vi "Setup.vi"(11 "Network Session Handler in":refnum<class "Network Session Handler.lvclass">) -> (0 "error out":errorcluster, 3 "Network Session Handler out":refnum<class "Network Session Handler.lvclass">)   [LabVIEW 2017, in "Network Interface.lvlib" / "Network Session Handler.lvclass"]
uses:
  <vilib>/gpm_packages/@cs/Network-sink/Source/Network Interface/Network Session Handler/Network Session Handler.lvclass
  <vilib>/gpm_packages/@cs/Network-sink/Source/Network Interface/Network Session Handler/Factory Loop Message Names ENUM.ctl
  <vilib>/gpm_packages/@cs/event-logger/Source/Composed Log/Types/Log Level.ctl
  <vilib>/gpm_packages/@cs/Network-sink/Source/Network Interface/Network Session Handler/Connection Handler.ctl
  <vilib>/gpm_packages/@cs/Network-sink/Source/Network Interface/Message Queue/Message Queue.lvclass
  <vilib>/gpm_packages/@cs/Network-sink/Source/Network Interface/Network Session Handler/Network Session Handler.lvclass/Network Session Handler.ctl
  <vilib>/gpm_packages/@cs/Network-sink/Source/Network Interface/Message Queue/Message Queue.lvclass/Message Queue.ctl
  <vilib>/gpm_packages/@cs/event-logger/Source/Composed Log/LoggerReference/LoggerReference.lvclass/LoggerReference.ctl
  f5036928-9ab8-417f-a1b8-cb07c5aeec2d.vi
  <vilib>/gpm_packages/@cs/Network-sink/Source/Network Interface/Message Queue/Protected Enqueue.vi
  <vilib>/gpm_packages/@cs/event-logger/Source/Composed Log/LoggerReference/Log.vi
  <vilib>/gpm_packages/@cs/event-logger/Source/Composed Log/LoggerReference/Get Valid Event Time.vi
  <vilib>/gpm_packages/@cs/event-logger/Source/Composed Log/LoggerReference/Remove Stale Logs.vi
  <vilib>/gpm_packages/@cs/event-logger/Source/Composed Log/Composed Log.lvlib
  <vilib>/Utility/Data Type/NI_Data Type.lvlib
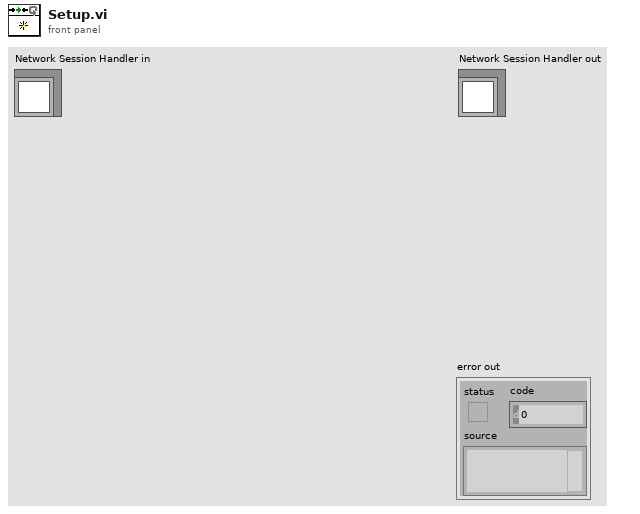
[diagram p1: front panel]
types:
  T1 = typedef "Network Interface.lvlib/Network Session Handler.lvclass/Connection Handler.ctl" = cluster{"ID":string, "Handler Queue":refnum<class "Message Queue.lvclass">}
  T2 = typedef "Composed Log.lvlib/Log Level.ctl" = enum16{"Debug", "Info", "Warning", "Error", "Critical"}
  T3 = typedef "Network Interface.lvlib/Network Session Handler.lvclass/Factory Loop Message Names ENUM.ctl" = enum16{"Create Connection", "Stop", "Assess Factory State"}
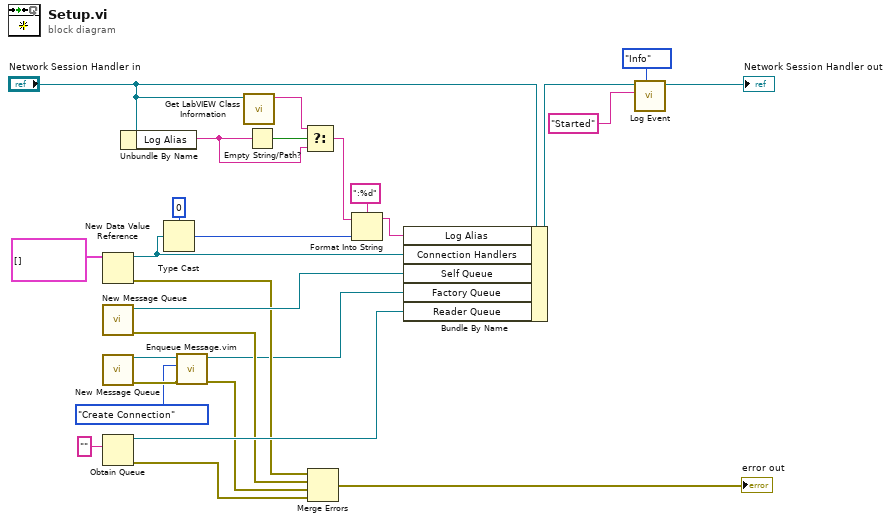
[diagram p0: block diagram]
diagram:
  n1 = New Data Value Reference(data value=T1[] []) -> (data value reference=w6:refnum<data-value>, error out=w24:errorcluster)  [unwired: 1 in]
  n2 = call <vilib>:"New Message Queue.vi"() -> ("error out"=w23:errorcluster, "Message Queue out"=w27:refnum<class "Message Queue.lvclass">)  [unwired: 10 in]
  n3 = call <vilib>:"New Message Queue.vi"() -> ("error out"=w18:errorcluster, "Message Queue out"=w20:refnum<class "Message Queue.lvclass">)  [unwired: 10 in]
  n4 = Obtain Queue(element data type="") -> (queue out=w25:refnum<queue>, error out=w22:errorcluster)  [unwired: 4 in, 1 out]
  n5 = Unbundle By Name("Network Session Handler in") -> ("Log Alias"=w9:string)
  n6 = Type Cast(type=0, x=w6) -> (*(type *) &x=w4:i32)
  n7 = call "Enqueue Message.vim"("error in (no error)"=w18, "Msg"=Factory_Loop_Message_Names_ENUM."Create Connection" ("Factory Message Names"), "Message Queue in"=w20) -> ("error out"=w17:errorcluster, "Message Queue out"=w19:refnum<class "Message Queue.lvclass">)  [unwired: 7 in]
  n8 = call <vilib>:"Get LabVIEW Class Information.vi"("Variant"="Network Session Handler in") -> ("LabVIEW Class File Name"=w7:string)  [unwired: 8 in, 2 out]
  n9 = Empty String/Path?(string/path=w9) -> (empty?=w10:bool)
  n10 = Select(t=w7, s=w10, f=w9) -> (s? t:f=w3:string)
  n11 = Merge Errors(w24, w23, w17, w22) -> (→"error out":errorcluster)
  n12 = Format Into String(format string=":%d", initial string=w3, w4) -> (resulting string=w1:string)  [unwired: 1 in, 1 out]
  n13 = Bundle By Name(cluster="Network Session Handler in", "Log Alias"=w1, "Connection Handlers"=w6, "Self Queue"=w27, "Factory Queue"=w19, "Reader Queue"=w25) -> (w14:refnum<class "Network Session Handler.lvclass">)
  n14 = call <vilib>:"Log Event.vi"("Event Level"=Log_Level."Info", "Event"="Started", "Network Session Handler in"=w14) -> ("Network Session Handler out"=→"Network Session Handler out":refnum<class "Network Session Handler.lvclass">)  [unwired: 7 in, 1 out]
